vi "Switch and DMM Configure.vi"(7 "Resistivity":T1, 8 "error in (no error)":errorcluster, 11 "VISA resource name":refnum<visa-resource-name>) -> (0 "error out":errorcluster, 3 "VISA resource name out":refnum<visa-resource-name>)   [LabVIEW 2016, in "Hall Effect Library.lvlib"]
uses:
  Hall Effect Library.lvlib
  Public/Controls/Resisitivity.ctl
  Global Variables/Test Settings.vi
  <instrlib>/Keithley 3706/Keithley 3706.lvlib
panel:
  out "resulting string":string
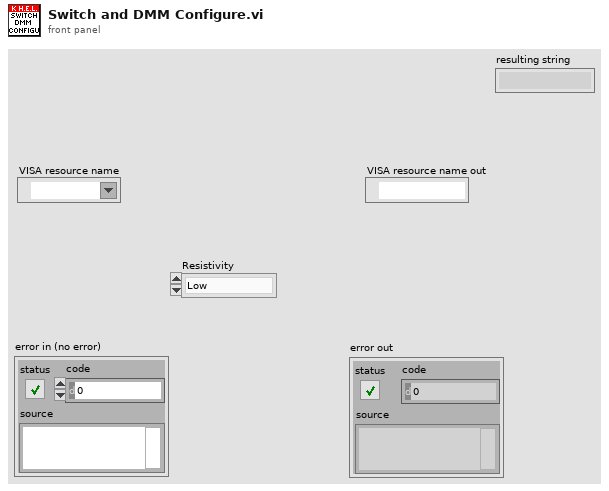
[diagram p1: front panel]
types:
  T1 = typedef "Hall Effect Library.lvlib/Resisitivity.ctl" = enum16{"Low", "High"}
  T2 = enum16{"BBM:Break Before Make", "MBB:Make Before Break", "OFF"}
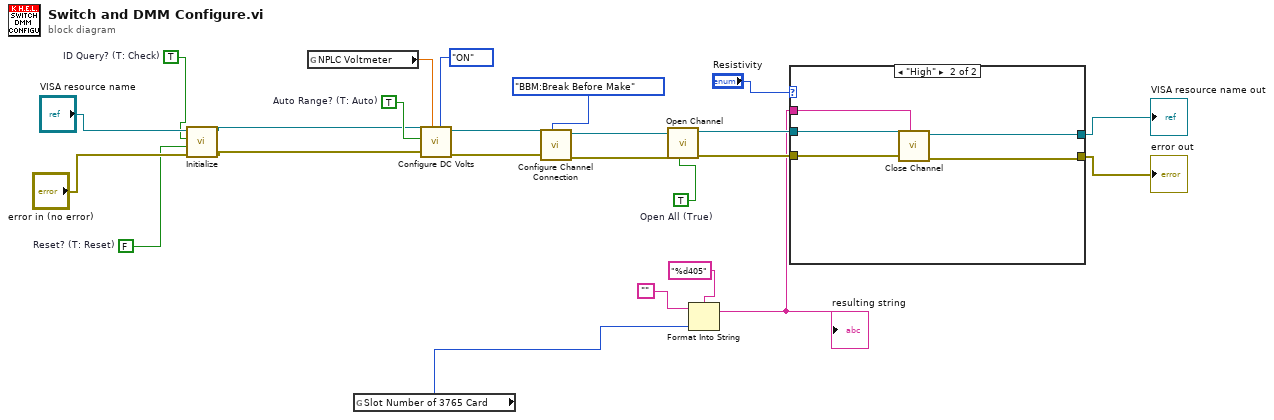
[diagram p0: block diagram]
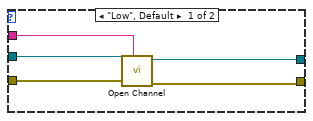
[diagram p2: hidden frame]
diagram:
  w10 = TRUE  # Open All (True)
  w20 = TRUE  # Auto Range? (T: Auto)
  w21 = FALSE  # Reset? (T: Reset)
  w22 = TRUE  # ID Query? (T: Check)
  n1 = call <instrlib>:"Initialize.vi"("error in (no error)"="error in (no error)", "Reset (True)"=w21, "ID Query (True)"=w22, "VISA resource name"="VISA resource name") -> ("error out"=w16:errorcluster, "VISA resource name out"=w17:refnum<visa-resource-name>)  [unwired: 6 in]
  n2 = global read "Test Settings.vi" "NPLC Voltmeter"() -> (w19:dbl)
  n3 = global read "Test Settings.vi" "Slot Number of 3765 Card"() -> (w4:u32)
  n4 = call <instrlib>:"Configure DC Volts.vi"("AutoZero"=enum16{"OFF", "ON", "ONCE"}."ON", "NPLC"=w19, "error in"=w16, "AutoRange  On"=w20, "VISA resource name"=w17) -> ("error out"=w14:errorcluster, "VISA resource name out"=w15:refnum<visa-resource-name>)  [unwired: 4 in, 1 out]
  n5 = call <instrlib>:"Configure Channel Connection.vi"("Channel Connect Rule"=T2."BBM:Break Before Make", "error in"=w14, "VISA resource name"=w15) -> ("error out"=w11:errorcluster, "VISA resource name out"=w12:refnum<visa-resource-name>)  [unwired: 7 in]
  n6 = call <instrlib>:"Open Channel.vi"("Open All (False)"=w10, "error in (no error)"=w11, "VISA resource name"=w12) -> ("error out"=w7:errorcluster, "VISA resource name out"=w8:refnum<visa-resource-name>)  [unwired: 7 in]
  n7 = Format Into String(format string="%d405", initial string="", w4) -> (resulting string=w2:string)  [unwired: 1 in, 1 out]
  "resulting string" <- w2
  n8 = case shown="\"High\"" "Resistivity" {
    tunnel: w8 -> [w29 w34]
    tunnel: w7 -> [w28 w33]
    tunnel: w2 -> [w27 w32]
    tunnel: [w26 w31] -> w6
    tunnel: [w25 w30] -> w5
    frame "Low", Default {
      n9 = call <instrlib>:"Open Channel.vi"("Channel List"=w27, "error in (no error)"=w28, "VISA resource name"=w29) -> ("error out"=w25:errorcluster, "VISA resource name out"=w26:refnum<visa-resource-name>)  [unwired: 7 in]
    }
    frame "High" {
      n10 = call <instrlib>:"Close Channel.vi"("Channel List"=w32, "error in (no error)"=w33, "VISA resource name"=w34) -> ("error out"=w30:errorcluster, "VISA resource name out"=w31:refnum<visa-resource-name>)  [unwired: 7 in]
    }
  }
  "VISA resource name out" <- w6
  "error out" <- w5
